vi "CANopenNMT.vi"(2 "error in":errorcluster, 3 "Mode":T1(ring), 4 "Node ID":u8, 5 "FPGA VI Reference In":refnum<k20>) -> (0 "error out":errorcluster, 1 "FPGA VI Reference Out":refnum<k20>)   [LabVIEW 2016]
doc: "This VI allows to change the CANopen network management state for all or a particular node."
uses:
  <vilib>/rvi/errors/niLvFpgaAdjustHostInterfaceError.vi
  <vilib>/Utility/error.llb/Error Cluster From Error Code.vi
  <vilib>/rvi/interface/nirviReadWriteControl/nirviReadWriteControl.xnode
  FPGA Bitfiles/EV-MCU_FPGATarget_CANEngine(FPGA)b_eM8Xz3qYJVA.lvbitx
  CAN_Engine(FPGA)_basic.vi
  NiFpgaLv.dll
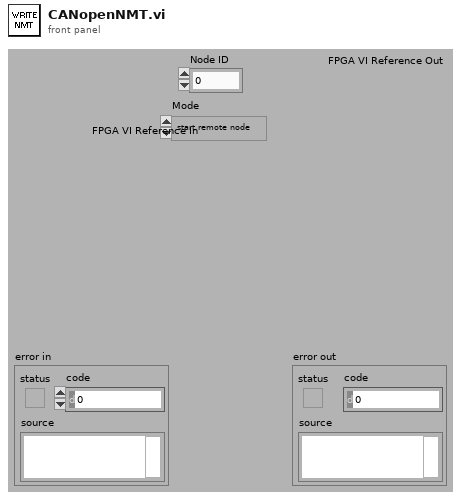
[diagram p1: front panel]
types:
  T1 = enum16{"start remote node", "stop remote node", "reset node", "reset communication", "enter preoperational"}
  T2 = cluster{"Data[0]":u8, "Data[1]":u8, "Data[2]":u8, "Data[3]":u8, "Data[4]":u8, "Data[5]":u8, "Data[6]":u8, "Data[7]":u8}
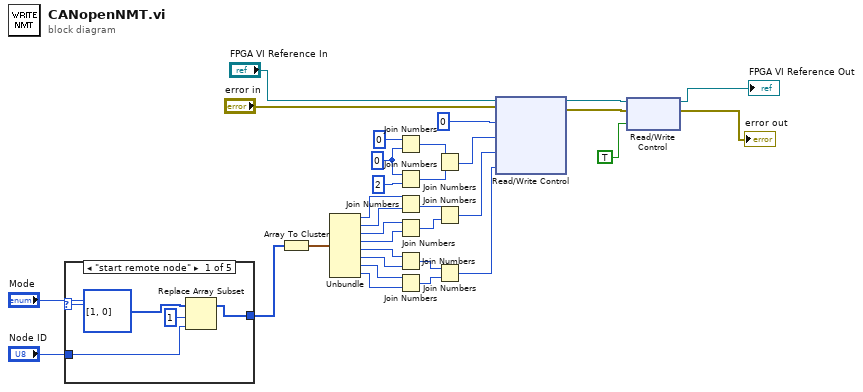
[diagram p0: block diagram]
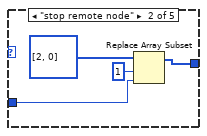
[diagram p2: hidden frame]
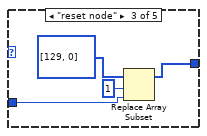
[diagram p3: hidden frame]
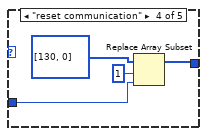
[diagram p4: hidden frame]
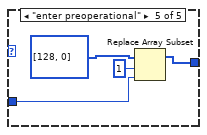
[diagram p5: hidden frame]
diagram:
  w11 = u8 0 ("lo")
  n1 = case shown="\"start remote node\"" "Mode" {
    tunnel: [w34 w37 w43 w45 w49] -> w13
    tunnel: "Node ID" -> [w33 w38 w41 w47 w50]
    frame "start remote node" {
      n2 = Replace Array Subset(array=u8[] [1, 0] ("Data"), new element=w33, index=1) -> (w34:u8[])
    }
    frame "stop remote node" {
      n3 = Replace Array Subset(array=u8[] [2, 0] ("Data"), new element=w38, index=1) -> (w37:u8[])
    }
    frame "reset node" {
      n4 = Replace Array Subset(array=u8[] [129, 0] ("Data"), new element=w41, index=1) -> (w43:u8[])
    }
    frame "reset communication" {
      n5 = Replace Array Subset(array=u8[] [130, 0] ("Data"), new element=w47, index=1) -> (w45:u8[])
    }
    frame "enter preoperational" {
      n6 = Replace Array Subset(array=u8[] [128, 0] ("Data"), new element=w50, index=1) -> (w49:u8[])
    }
  }
  n7 = Array To Cluster(array=w13) -> (cluster=w14:T2)
  n8 = Unbundle(w14) -> ("Data[0]"=w18:u8, "Data[1]"=w19:u8, "Data[2]"=w23:u8, "Data[3]"=w20:u8, "Data[4]"=w21:u8, "Data[5]"=w22:u8, "Data[6]"=w24:u8, "Data[7]"=w25:u8)
  n9 = Join Numbers(hi=u8 0, lo=w11) -> ((hi.lo)=w9:u16)
  n10 = Join Numbers(hi=w11, lo=u8 2) -> ((hi.lo)=w10:u16)
  n11 = Join Numbers(hi=w18, lo=w19) -> ((hi.lo)=w15:u16)
  n12 = Join Numbers(hi=w23, lo=w20) -> ((hi.lo)=w26:u16)
  n13 = Join Numbers(hi=w21, lo=w22) -> ((hi.lo)=w16:u16)
  n14 = Join Numbers(hi=w24, lo=w25) -> ((hi.lo)=w17:u16)
  n15 = Join Numbers(hi=w9, lo=w10) -> ((hi.lo)=w6:u32)
  n16 = Join Numbers(hi=w15, lo=w26) -> ((hi.lo)=w5:u32)
  n17 = Join Numbers(hi=w16, lo=w17) -> ((hi.lo)=w4:u32)
  n18 = xnode "Read/Write Control"("FPGA VI Reference In"="FPGA VI Reference In", "error in"="error in", "U32 Out 3"=u32 0 ("ArbitrationId"), "U32 Out 4"=w6, "U32 Out 5"=w5, "U32 Out 6"=w4) -> ("FPGA VI Reference Out"=w30:refnum<k20>, "error out"=w29:errorcluster)
  n19 = xnode "Read/Write Control"("FPGA VI Reference In"=w30, "error in"=w29, "Write"=TRUE) -> ("FPGA VI Reference Out"=→"FPGA VI Reference Out":refnum<k20>, "error out"=→"error out":errorcluster)
